vi "Read Ref.vi"(8 "error in (no error)":errorcluster, 11 "BetterDropOp in":refnum<class "BetterDropOp.lvclass">) -> (0 "error out":errorcluster, 2 "Ref":refnum<vi>, 3 "BetterDropOp out":refnum<class "BetterDropOp.lvclass">)   [LabVIEW 2020, in "BetterDragAndDrop.lvlib" / "BetterDropOp.lvclass"]
uses:
  BetterDropOp.lvclass
  BetterDropOp.lvclass/BetterDropOp.ctl
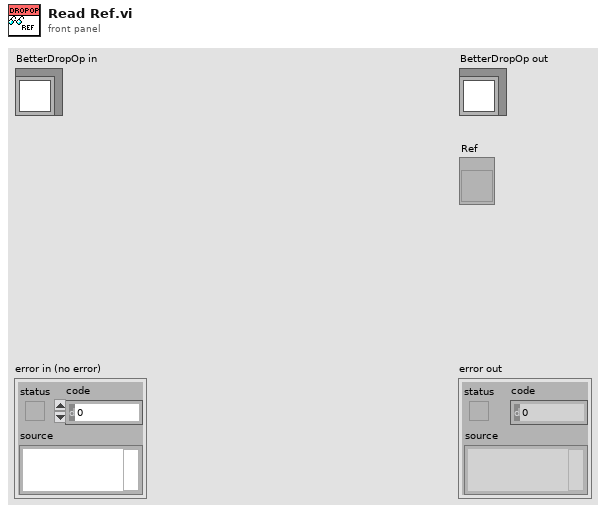
[diagram p1: front panel]
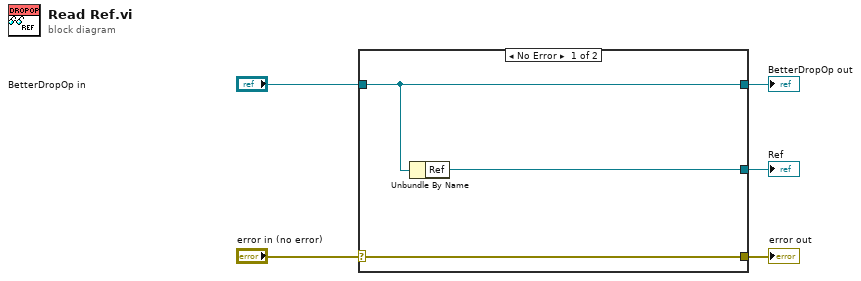
[diagram p0: block diagram]
diagram:
  n1 = case shown="No Error" "error in (no error)" {
    selector: "error in (no error)" -> [w8 w9]
    tunnel: [w8 w9] -> w4
    tunnel: [w7 w10] -> w2
    tunnel: "BetterDropOp in" -> [w7 w10]
    tunnel: [w6 _] -> w1
    frame No Error {
      n2 = Unbundle By Name(w7) -> ("Ref"=w6:refnum<vi>)
    }
    frame Error {
    }
  }
  "error out" <- w4
  "BetterDropOp out" <- w2
  "Ref" <- w1
